vi "Get position.vi"(6 "Motor params":T1 {"Tipo de paso" items=["Medio paso", "Paso completo"]; "Dirección" items=["Izquierda", "Derecha"]; "Tipo" items=["Izquierda", "Derecha"]}, 7 "mm/step":dbl=0.0025 format="%#_13g", 8 "error in (no error)":errorcluster, 10 "Recibo de Datos":string, 11 "Position":dbl) -> (0 "error out":errorcluster, 3 "Position out":dbl)   [LabVIEW 2020, in "Control de MaP.lvlib"]
uses:
  Controls/Command to motor.ctl
  Control de MaP.lvlib
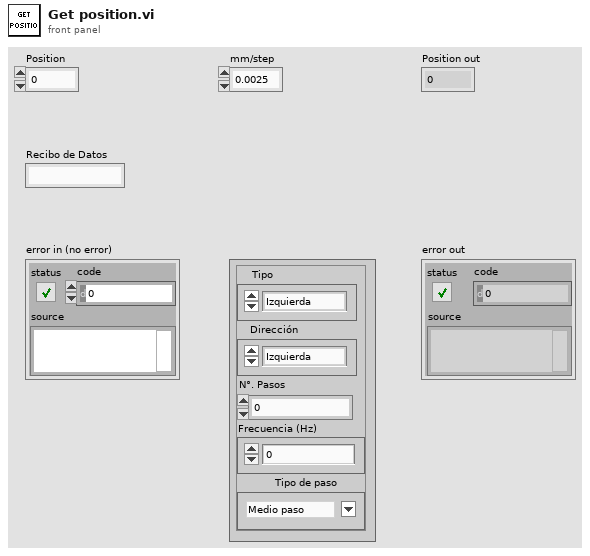
[diagram p1: front panel]
types:
  T1 = typedef "Control de MaP.lvlib/Command to motor.ctl" = cluster{"Tipo":u8, "Dirección":u8, "N°. Pasos":u16, "Frecuencia (Hz)":u8, "Tipo de paso":u8}
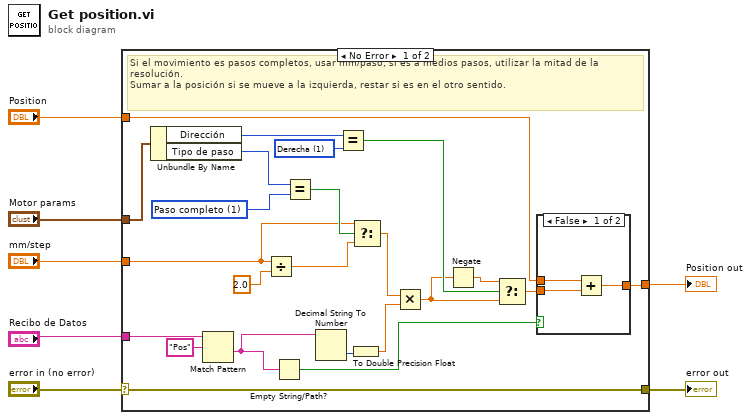
[diagram p0: block diagram]
diagram:
  n1 = case shown="No Error" "error in (no error)" {
    selector: "error in (no error)" -> [w26 w36]
    tunnel: [w15 w35] -> w7
    tunnel: "Position" -> [w13 w35]
    tunnel: "Recibo de Datos" -> [w28 _]
    tunnel: [w26 w36] -> w3
    tunnel: "Motor params" -> [w25 _]
    tunnel: "mm/step" -> [w12 _]
    frame No Error {
      w19 = u8 1 items=["Izquierda", "Derecha"] ("Dirección")
      w23 = u8 1 items=["Medio paso", "Paso completo"] ("Tipo de paso")
      # "Si el movimiento es pasos completos, usar mm/paso, si es a medios pasos, utilizar la mitad de la resolución.\nSumar a la posición si se mueve a la izquierda, restar si es en el otro sentido."
      n2 = Unbundle By Name(w25) -> ("Dirección"=w20:u8, "Tipo de paso"=w24:u8)
      n3 = Match Pattern(string=w28, regular expression="Pos") -> (after substring=w9:string)  [unwired: 1 in, 3 out]
      n4 = Divide(x=w12, y=2.0) -> (x/y=w10:dbl)
      n5 = Empty String/Path?(string/path=w9) -> (empty?=w8:bool)
      n6 = Equal?(x=w24, y=w23) -> (x = y?=w22:bool)
      n7 = Decimal String To Number(string=w9) -> (number=w30:i32)  [unwired: 2 in, 1 out]
      n8 = Equal?(x=w20, y=w19) -> (x = y?=w18:bool)
      n9 = To Double Precision Float(number=w30) -> (double precision float=w27:dbl)
      n10 = Select(t=w12, s=w22, f=w10) -> (s? t:f=w21:dbl)
      n11 = Multiply(x=w21, y=w27) -> (x*y=w16:dbl)
      n12 = Negate(x=w16) -> (-x=w17:dbl)
      n13 = Select(t=w17, s=w18, f=w16) -> (s? t:f=w14:dbl)
      n14 = case shown="False" w8 {
        tunnel: [w33 w34] -> w15
        tunnel: w14 -> [w32 _]
        tunnel: w13 -> [w31 w34]
        frame False {
          n15 = Add(x=w31, y=w32) -> (x+y=w33:dbl)
        }
        frame True {
        }
      }
    }
    frame Error {
    }
  }
  "Position out" <- w7
  "error out" <- w3
